vi "Shooter logic.vi"(0 "Low Pressure?":bool, 1 "Fire Main":bool, 2 "Fire 3":bool, 3 "Fire 2":bool, 5 "Grabber Button":bool, 6 "Time Between Open and Shoot":u32=250, 7 "Arms Up button":bool, 8 "Release to Retract":u32=750, 9 "Arms Down Button":bool, 10 "Arms up and down":dbl) -> ()   [LabVIEW 2013]
uses:
  <vilib>/Rock Robotics/WPI/Solenoid/WPI_SolenoidValue.ctl
  <vilib>/Rock Robotics/WPI/Solenoid/WPI_SolenoidSetEnum.vi
  Robot Global Data.vi
panel:
  in  "Arm State":enum16{"Close Arms", "Open Arms"}(ring)
  in  "Launcher State":T1(ring)
  out "Tick":u32
  out "Retract Position":T2
  out "Shooter Position":T2
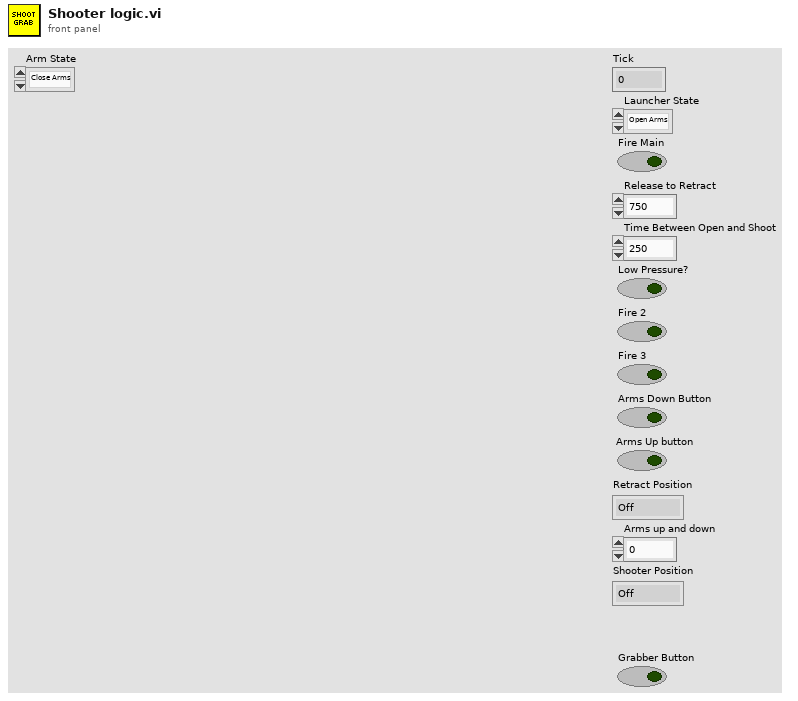
[diagram p1: front panel]
types:
  T1 = enum16{"Open Arms", "Arms Open", "Shoot", "Out", "Retract"}
  T2 = typedef "WPI_SolenoidValue.ctl" = enum16{"Off", "On", "Forward", "Reverse"}
  T3 = typedef "WPI_SolenoidDevRef.ctl" = cluster{"DevStatus":errorcluster, "Solenoid Module":T4, "Forward Solenoid Channel":T5, "Reverse Solenoid Channel":T5}
  T4 = typedef "FPGA_TypedefSolenoidModule.ctl" = enum16{"Solenoid Module 1", "Solenoid Module 2"}
  T5 = typedef "WPI_SolenoidChannel.ctl" = enum8{"Solenoid 1", "Solenoid 2", "Solenoid 3", "Solenoid 4", "Solenoid 5", "Solenoid 6", "Solenoid 7", "Solenoid 8", "Invalid"}
  T6 = typedef "WPI_DigitalInputDevRef.ctl" = cluster{"DevStatus":errorcluster, "DIO Channel":T7, "Digital Module":T8}
  T7 = typedef "FPGA_DIOChannel.ctl" = enum8{"DIO 1", "DIO 2", "DIO 3", "DIO 4", "DIO 5", "DIO 6", "DIO 7", "DIO 8", "DIO 9", "DIO 10", "DIO 11", "DIO 12", "DIO 13", "DIO 14", "Invalid"}
  T8 = typedef "FPGA_TypedefDigitalModule.ctl" = enum16{"Digital Module 1", "Digital Module 2"}
  T9 = typedef "WPI_MotorControlDeviceRef.ctl" = cluster{"DeviceStatus":errorcluster, "Type":enum16{"PWM", "CAN"}, "PWM":cluster{"Digital Module":T8, "PWM Channel":T10, "DeadBand":T11}, "CAN":cluster{"Device Number":u8, "Control Mode":T12, "Semaphore":T13, "Max Vout":dbl}, "Invert":bool, "TransformRef":T14, "InvTransformRef":T14}
  T10 = typedef "FPGA_DIOPWMChannel.ctl" = enum8{"PWM 1", "PWM 2", "PWM 3", "PWM 4", "PWM 5", "PWM 6", "PWM 7", "PWM 8", "PWM 9", "PWM 10", "Invalid"}
  T11 = typedef "WPI_PWMDeadband.ctl" = cluster{"Name":string, "maxPositivePwm":i32, "minPositivePwm":i32, "centerPwm":i32, "maxNegativePwm":i32, "minNegativePwm":i32, "angularRange":u16}
  T12 = typedef "WPI_CANJaguar_ControlMode.ctl" = enum8{"Percent VBus", "Current", "Speed", "Position", "Voltage"}
  T13 = typedef "Semaphore RefNum" = refnum<k1>
  T14 = typedef "WPI_PWMTransform_ConPane.ctl" = refnum<vi>
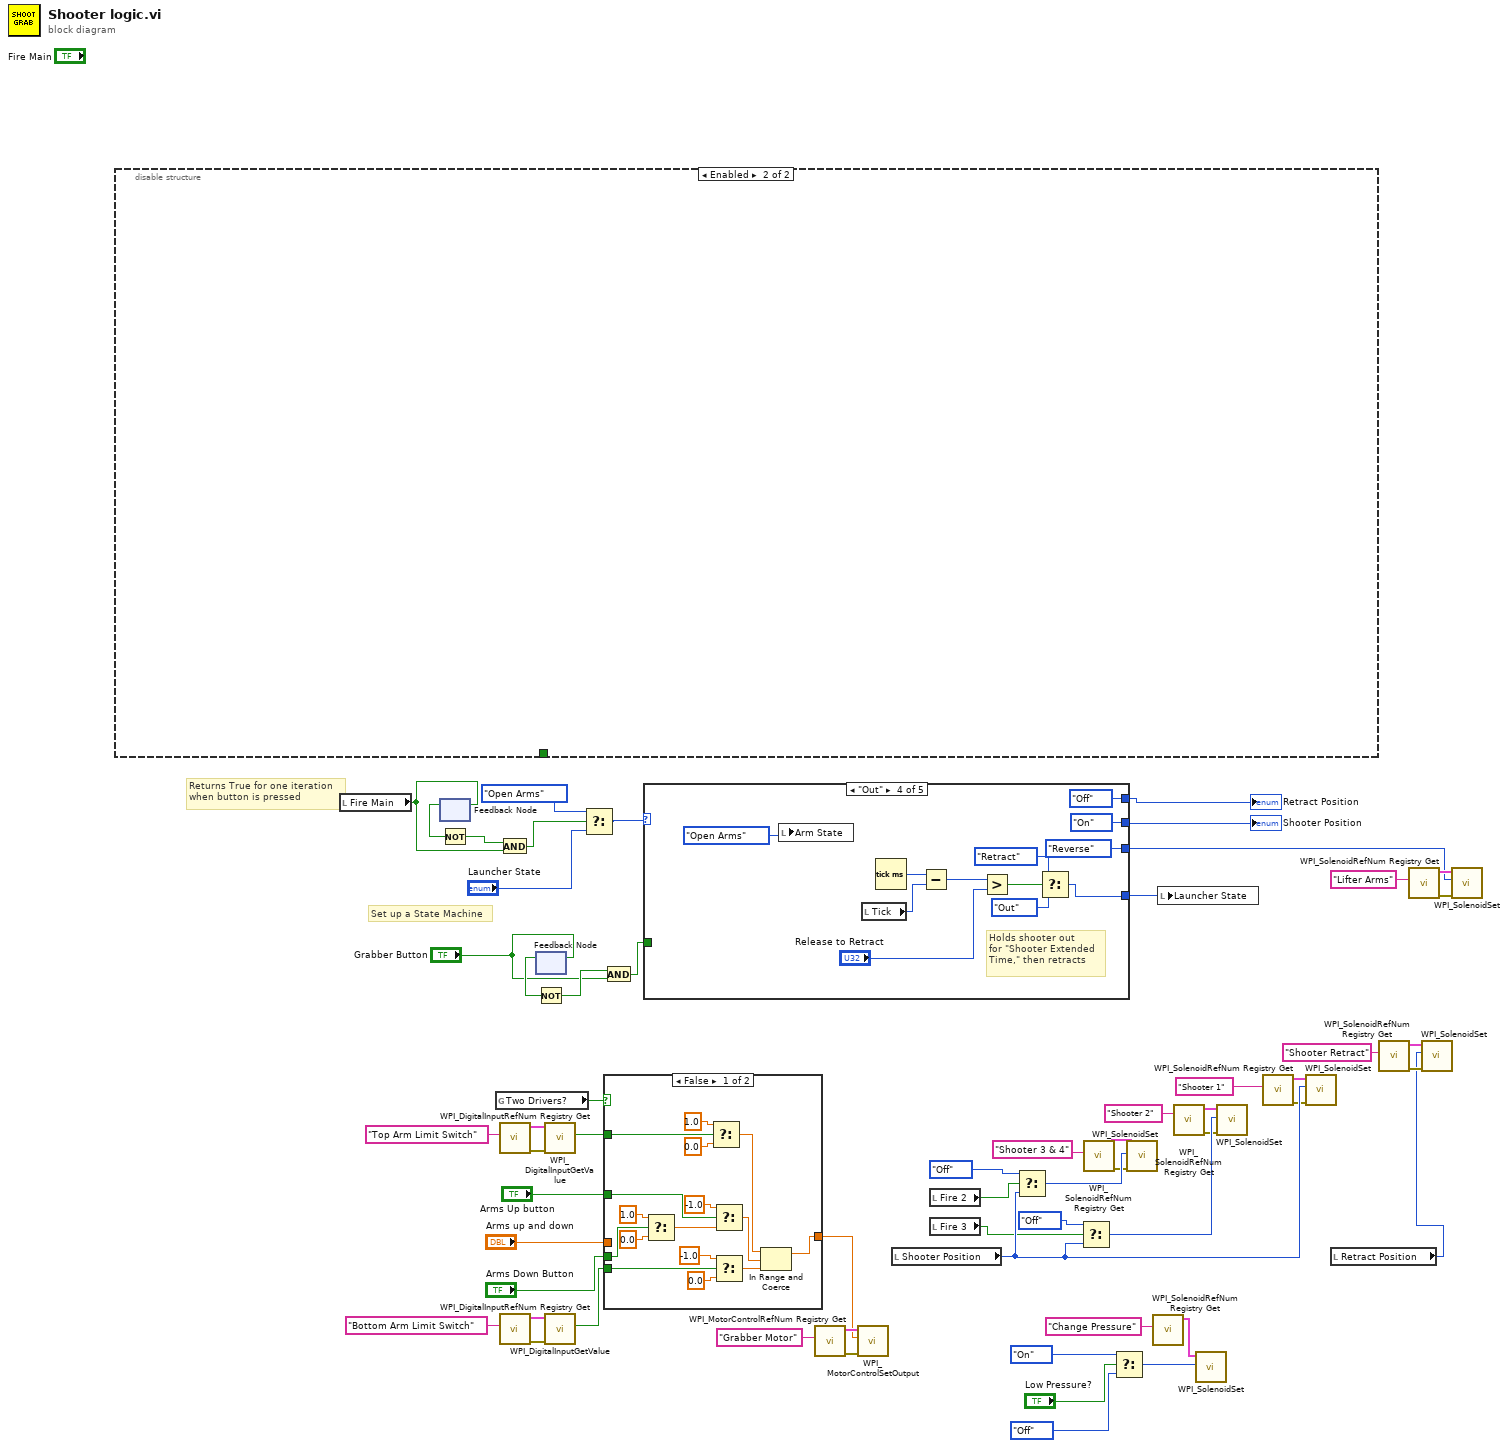
[diagram p0: block diagram]
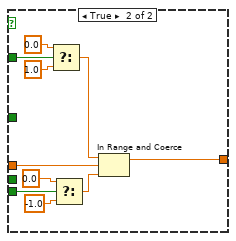
[diagram p2: hidden frame]
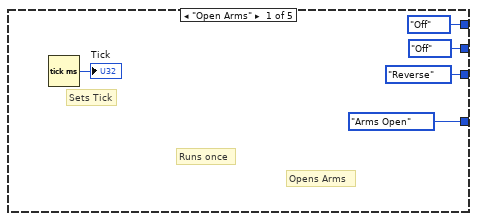
[diagram p3: hidden frame]
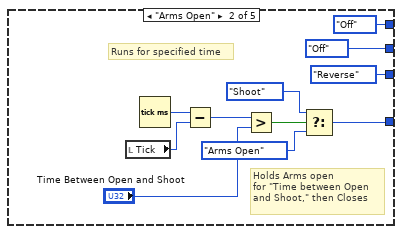
[diagram p4: hidden frame]
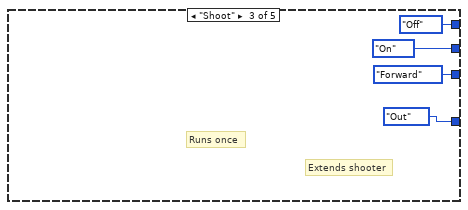
[diagram p5: hidden frame]
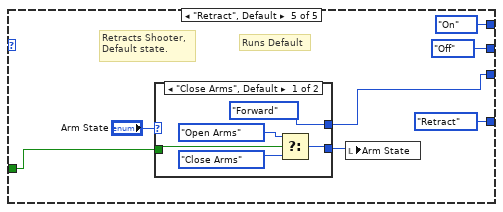
[diagram p6: hidden frame]
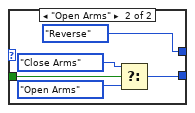
[diagram p7: hidden frame]
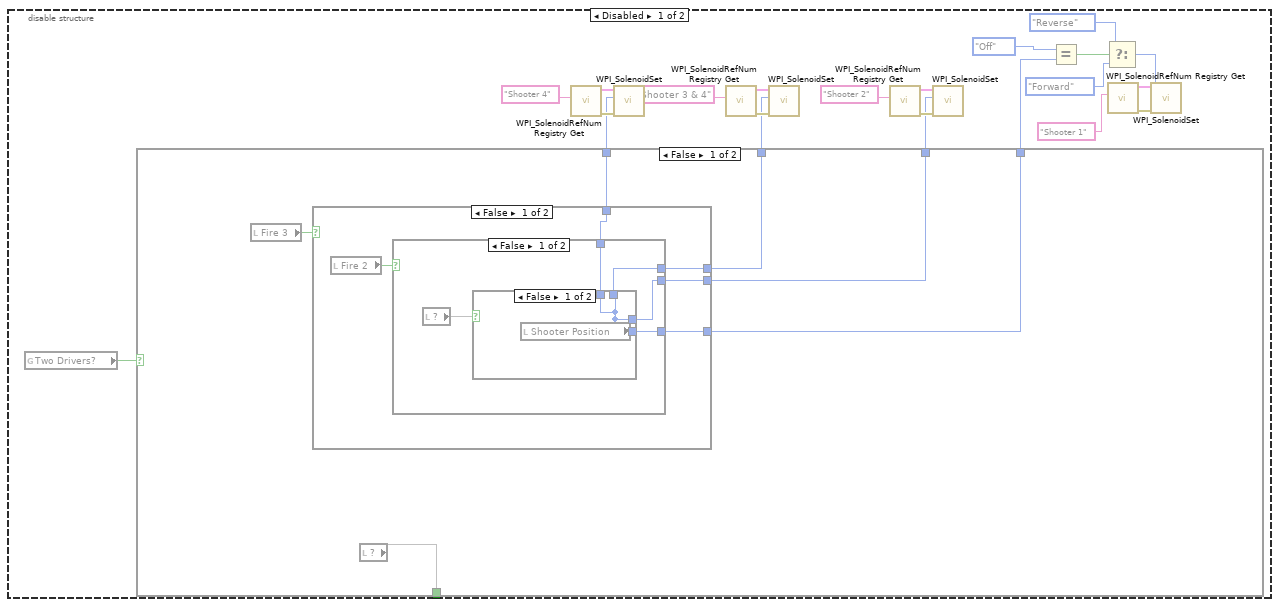
[diagram p8: hidden frame]
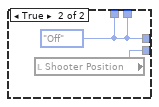
[diagram p9: hidden frame]
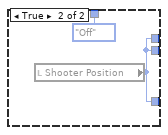
[diagram p10: hidden frame]
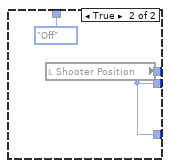
[diagram p11: hidden frame]
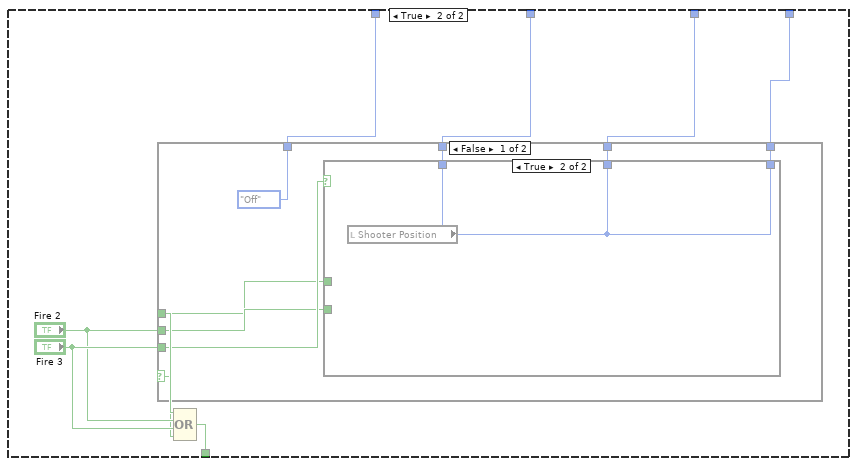
[diagram p12: hidden frame]
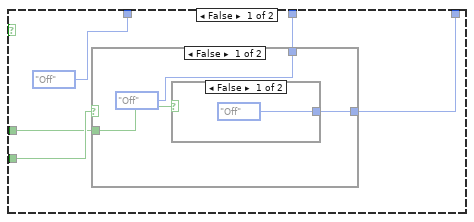
[diagram p13: hidden frame]
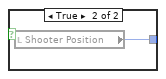
[diagram p14: hidden frame]
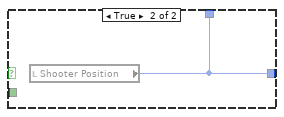
[diagram p15: hidden frame]
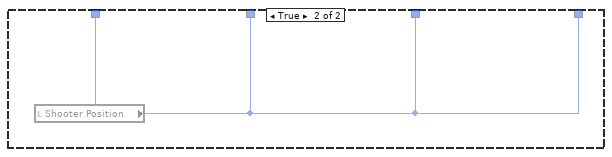
[diagram p16: hidden frame]
diagram:
  # "Set up a State Machine"
  # "Returns True for one iteration\nwhen button is pressed"
  n1 = disable-structure shown="Enabled" {
    disable-tunnel: [w83 _] -> _
    frame Disabled {
      n2 = global read "Robot Global Data.vi" "Two Drivers?"() -> (w82:bool)
      n3 = case shown="False" w82 {
        tunnel: [w89 w115] -> w83
        tunnel: [w84 w110] -> w64
        tunnel: [w87 w109] -> w63
        tunnel: [w86 w108] -> w62
        tunnel: [w85 w107] -> w61
        frame False {
          n4 = local read "Fire 3"() -> (w88:bool)
          n5 = case shown="False" w88 {
            tunnel: [w93 w106] -> w87
            tunnel: [w92 w106] -> w86
            tunnel: [w91 w106] -> w85
            tunnel: [w90 WPI_SolenoidValue."Off" ("Position")] -> w84
            frame False {
              n6 = local read "Fire 2"() -> (w94:bool)
              n7 = case shown="False" w94 {
                tunnel: [w96 w104] -> w93
                tunnel: [w97 w104] -> w92
                tunnel: [w98 w104] -> w91
                tunnel: [w95 WPI_SolenoidValue."Off" ("Position")] -> w90
                frame False {
                  n8 = local read item#-1() -> (w99)
                  n9 = case shown="False" w99 {
                    tunnel: [w100 w102] -> w98
                    tunnel: [w100 w101] -> w97
                    tunnel: [w100 w101] -> w96
                    tunnel: [w100 w101] -> w95
                    frame False {
                      n10 = local read "Shooter Position"() -> (w100:T2)
                    }
                    frame True {
                      w101 = WPI_SolenoidValue."Off" ("Position")
                      n11 = local read "Shooter Position"() -> (w102:T2)
                    }
                  }
                }
                frame True {
                  n12 = local read "Shooter Position"() -> (w104:T2)
                }
              }
            }
            frame True {
              n13 = local read "Shooter Position"() -> (w106:T2)
            }
          }
          n14 = local read item#-1() -> (w89)
        }
        frame True {
          n15 = Compound Arithmetic op=OR("Fire 2", "Fire 3") -> (w115:bool, w112:bool, w111:bool)
          n16 = case shown="False" w111 {
            tunnel: [w118 w135] -> w107
            tunnel: [w119 w135] -> w108
            tunnel: [w120 w135] -> w109
            tunnel: [WPI_SolenoidValue."Off" ("Value") w135] -> w110
            tunnel: "Fire 3" -> [w121 _]
            tunnel: "Fire 2" -> [w117 _]
            tunnel: w112 -> [w116 _]
            frame False {
              n17 = case shown="True" w121 {
                tunnel: [WPI_SolenoidValue."Off" ("Value") w134] -> w120
                tunnel: [w127 w134] -> w119
                tunnel: [w126 w134] -> w118
                tunnel: w117 -> [w125 _]
                tunnel: w116 -> [w124 _]
                frame False {
                  n18 = case shown="False" w125 {
                    tunnel: [WPI_SolenoidValue."Off" ("Value") w133] -> w127
                    tunnel: [w128 w133] -> w126
                    tunnel: w124 -> [w129 _]
                    frame False {
                      n19 = case shown="False" w129 {
                        tunnel: [WPI_SolenoidValue."Off" ("Value") w132] -> w128
                        frame False {
                        }
                        frame True {
                          n20 = local read "Shooter Position"() -> (w132:T2)
                        }
                      }
                    }
                    frame True {
                      n21 = local read "Shooter Position"() -> (w133:T2)
                    }
                  }
                }
                frame True {
                  n22 = local read "Shooter Position"() -> (w134:T2)
                }
              }
            }
            frame True {
              n23 = local read "Shooter Position"() -> (w135:T2)
            }
          }
        }
      }
      n24 = call <vilib>:"WPI_SolenoidRefNum Registry Get.vi"("refnum name"="Shooter 4") -> ("error out"=w74:errorcluster, "SolenoidDevRef"=w75:T3)  [unwired: 9 in]
      n25 = call-poly <vilib>:"WPI_SolenoidSet.vi"("error in (no error)"=w74, "Value"=w64, "SolenoidDevRef"=w75) -> ()  [unwired: 7 in, 2 out]
      n26 = call <vilib>:"WPI_SolenoidRefNum Registry Get.vi"("refnum name"="Shooter 3 & 4") -> ("error out"=w77:errorcluster, "SolenoidDevRef"=w76:T3)  [unwired: 9 in]
      n27 = call-poly <vilib>:"WPI_SolenoidSet.vi"("error in (no error)"=w77, "Value"=w63, "SolenoidDevRef"=w76) -> ()  [unwired: 7 in, 2 out]
      n28 = call <vilib>:"WPI_SolenoidRefNum Registry Get.vi"("refnum name"="Shooter 2") -> ("error out"=w80:errorcluster, "SolenoidDevRef"=w81:T3)  [unwired: 9 in]
      n29 = call-poly <vilib>:"WPI_SolenoidSet.vi"("error in (no error)"=w80, "Value"=w62, "SolenoidDevRef"=w81) -> ()  [unwired: 7 in, 2 out]
      n30 = Equal?(x=WPI_SolenoidValue."Off" ("y"), y=w61) -> (x = y?=w67:bool)
      n31 = Select(t=WPI_SolenoidValue."Reverse" ("y"), s=w67, f=WPI_SolenoidValue."Forward" ("y")) -> (s? t:f=w70:T2)
      n32 = call <vilib>:"WPI_SolenoidRefNum Registry Get.vi"("refnum name"="Shooter 1") -> ("error out"=w66:errorcluster, "SolenoidDevRef"=w65:T3)  [unwired: 9 in]
      n33 = call-poly <vilib>:"WPI_SolenoidSet.vi"("error in (no error)"=w66, "Value"=w70, "SolenoidDevRef"=w65) -> ()  [unwired: 7 in, 2 out]
    }
    frame Enabled {
    }
  }
  n34 = local read "Fire Main"() -> (w20:bool)
  n35 = feedback #1() -> (w21:bool)  [unwired: 1 in]
  n36 = feedback-in #1(w20) -> ()
  n37 = Not(x=w21) -> (.not. x?=w22:bool)
  n38 = global read "Robot Global Data.vi" "Two Drivers?"() -> (w15:bool)
  n39 = And(x=w22, y=w20) -> (x .and. y?=w17:bool)
  n40 = call <vilib>:"WPI_DigitalInputRefNum Registry Get.vi"("refnum name"="Top Arm Limit Switch") -> ("error out"=w29:errorcluster, "DigitalInputDevRef"=w30:T6)  [unwired: 9 in]
  n41 = call <vilib>:"WPI_DigitalInputRefNum Registry Get.vi"("refnum name"="Bottom Arm Limit Switch") -> ("error out"=w26:errorcluster, "DigitalInputDevRef"=w27:T6)  [unwired: 9 in]
  n42 = feedback #2() -> (w4:bool)  [unwired: 1 in]
  n43 = feedback-in #2("Grabber Button") -> ()
  n44 = Not(x=w4) -> (.not. x?=w3:bool)
  n45 = call <vilib>:"WPI_DigitalInputGetValue.vi"("error in (no error)"=w29, "DigitalInputDevRef"=w30) -> ("Value"=w14:bool)  [unwired: 7 in, 2 out]
  n46 = call <vilib>:"WPI_DigitalInputGetValue.vi"("error in (no error)"=w26, "DigitalInputDevRef"=w27) -> ("Value"=w13:bool)  [unwired: 7 in, 2 out]
  n47 = Select(t=T1."Open Arms", s=w17, f="Launcher State") -> (s? t:f=w19:T1)
  n48 = And(x=w3, y="Grabber Button") -> (x .and. y?=w1:bool)
  n49 = case shown="False" w15 {
    tunnel: w14 -> [w143 w161]
    tunnel: w13 -> [w139 w157]
    tunnel: [w136 w153] -> w10
    tunnel: "Arms Up button" -> [w138 _]
    tunnel: "Arms Down Button" -> [w137 _]
    tunnel: "Arms up and down" -> [_ w152]
    frame False {
      n50 = Select(t=1.0, s=w137, f=0.0) -> (s? t:f=w149:dbl)
      n51 = Select(t=1.0, s=w143, f=0.0) -> (s? t:f=w144:dbl)
      n52 = Select(t=-1.0, s=w138, f=w149) -> (s? t:f=w147:dbl)
      n53 = Select(t=-1.0, s=w139, f=0.0) -> (s? t:f=w140:dbl)
      n54 = In Range and Coerce(upper limit=w144, x=w147, lower limit=w140) -> (coerced(x)=w136:dbl)  [unwired: 1 out]
    }
    frame True {
      n55 = Select(t=0.0, s=w161, f=1.0) -> (s? t:f=w160:dbl)
      n56 = Select(t=0.0, s=w157, f=-1.0) -> (s? t:f=w156:dbl)
      n57 = In Range and Coerce(upper limit=w160, x=w152, lower limit=w156) -> (coerced(x)=w153:dbl)  [unwired: 1 out]
    }
  }
  n58 = case shown="\"Out\"" w19 {
    tunnel: [WPI_SolenoidValue."Off" ("Value") WPI_SolenoidValue."Off" ("Value") WPI_SolenoidValue."On" ("Value") WPI_SolenoidValue."On" ("Value") WPI_SolenoidValue."Off" ("Value")] -> w7
    tunnel: [T1."Arms Open" ("Launcher State") w168 T1."Out" ("Launcher State") w186 T1."Retract" ("Launcher State")] -> w6
    tunnel: [WPI_SolenoidValue."Reverse" ("Arm Position") WPI_SolenoidValue."Reverse" ("Arm Position") WPI_SolenoidValue."Forward" ("Arm Position") WPI_SolenoidValue."Reverse" ("Arm Position") w196] -> w5
    tunnel: [WPI_SolenoidValue."Off" ("Value") WPI_SolenoidValue."Off" ("Value") WPI_SolenoidValue."Off" ("Value") WPI_SolenoidValue."Off" ("Value") WPI_SolenoidValue."On" ("Value")] -> w8
    tunnel: w1 -> [_ _ _ _ w197]
    frame "Open Arms" {
      # "Opens Arms"
      # "Runs once"
      # "Sets Tick"
      n59 = Tick Count (ms)() -> (millisecond timer value=→"Tick":u32)
    }
    frame "Arms Open" {
      # "Runs for specified time"
      # "Holds Arms open\nfor \"Time between Open\nand Shoot,\" then Closes"
      n60 = local read "Tick"() -> (w176:u32)
      n61 = Tick Count (ms)() -> (millisecond timer value=w177:u32)
      n62 = Subtract(x=w177, y=w176) -> (x-y=w175:u32)
      n63 = Greater?(x=w175, y="Time Between Open and Shoot") -> (0:w174:bool)
      n64 = Select(t=T1."Shoot" ("Launcher State"), s=w174, f=T1."Arms Open" ("Launcher State")) -> (s? t:f=w168:T1)
    }
    frame "Shoot" {
      # "Runs once"
      # "Extends shooter"
    }
    frame "Out" {
      # "Holds shooter out\nfor \"Shooter Extended\nTime,\" then retracts"
      n65 = local write "Arm State"(enum16{"Close Arms", "Open Arms"}."Open Arms" ("Arm State")) -> ()
      n66 = local read "Tick"() -> (w192:u32)
      n67 = Tick Count (ms)() -> (millisecond timer value=w193:u32)
      n68 = Subtract(x=w193, y=w192) -> (x-y=w191:u32)
      n69 = Greater?(x=w191, y="Release to Retract") -> (0:w190:bool)
      n70 = Select(t=T1."Retract" ("Launcher State"), s=w190, f=T1."Out" ("Launcher State")) -> (s? t:f=w186:T1)
    }
    frame "Retract", Default {
      # "Runs Default"
      # "Retracts Shooter, \nDefault state."
      n71 = case shown="\"Close Arms\", Default" "Arm State" {
        tunnel: w197 -> [w201 w206]
        tunnel: [WPI_SolenoidValue."Forward" ("Value") WPI_SolenoidValue."Reverse" ("Value")] -> w196
        tunnel: [w202 w207] -> w194
        frame "Close Arms", Default {
          n72 = Select(t=enum16{"Close Arms", "Open Arms"}."Open Arms", s=w201, f=enum16{"Close Arms", "Open Arms"}."Close Arms") -> (s? t:f=w202:enum16{"Close Arms", "Open Arms"})
        }
        frame "Open Arms" {
          n73 = Select(t=enum16{"Close Arms", "Open Arms"}."Close Arms", s=w206, f=enum16{"Close Arms", "Open Arms"}."Open Arms") -> (s? t:f=w207:enum16{"Close Arms", "Open Arms"})
        }
      }
      n74 = local write "Arm State"(w194) -> ()
    }
  }
  "Shooter Position" <- w7
  "Retract Position" <- w8
  n75 = call <vilib>:"WPI_MotorControlRefNum Registry Get.vi"("refnum name"="Grabber Motor") -> ("error out"=w25:errorcluster, "MotorControlDevRef"=w24:T9)  [unwired: 9 in]
  n76 = call <vilib>:"WPI_MotorControlSetOutput.vi"("error in (no error)"=w25, "Output"=w10, "MotorControlDevRef"=w24) -> ()  [unwired: 6 in, 3 out]
  n77 = local read "Shooter Position"() -> (w57:T2)
  n78 = local read "Fire 2"() -> (w52:bool)
  n79 = local read "Fire 3"() -> (w48:bool)
  n80 = Select(t=WPI_SolenoidValue."Off", s=w52, f=w57) -> (s? t:f=w53:T2)
  n81 = Select(t=WPI_SolenoidValue."Off", s=w48, f=w57) -> (s? t:f=w49:T2)
  n82 = call <vilib>:"WPI_SolenoidRefNum Registry Get.vi"("refnum name"="Shooter 3 & 4") -> ("error out"=w43:errorcluster, "SolenoidDevRef"=w44:T3)  [unwired: 9 in]
  n83 = Select(t=WPI_SolenoidValue."On", s="Low Pressure?", f=WPI_SolenoidValue."Off" ("t")) -> (s? t:f=w34:T2)
  n84 = call-poly <vilib>:"WPI_SolenoidSet.vi"("error in (no error)"=w43, "Value"=w53, "SolenoidDevRef"=w44) -> ()  [unwired: 7 in, 2 out]
  n85 = call <vilib>:"WPI_SolenoidRefNum Registry Get.vi"("refnum name"="Change Pressure") -> ("SolenoidDevRef"=w38:T3)  [unwired: 9 in, 1 out]
  n86 = local write "Launcher State"(w6) -> ()
  n87 = call <vilib>:"WPI_SolenoidRefNum Registry Get.vi"("refnum name"="Shooter 2") -> ("error out"=w40:errorcluster, "SolenoidDevRef"=w39:T3)  [unwired: 9 in]
  n88 = call-poly <vilib>:"WPI_SolenoidSet.vi"("Value"=w34, "SolenoidDevRef"=w38) -> ()  [unwired: 8 in, 2 out]
  n89 = call-poly <vilib>:"WPI_SolenoidSet.vi"("error in (no error)"=w40, "Value"=w49, "SolenoidDevRef"=w39) -> ()  [unwired: 7 in, 2 out]
  n90 = call <vilib>:"WPI_SolenoidRefNum Registry Get.vi"("refnum name"="Shooter 1") -> ("error out"=w46:errorcluster, "SolenoidDevRef"=w47:T3)  [unwired: 9 in]
  n91 = call-poly <vilib>:"WPI_SolenoidSet.vi"("error in (no error)"=w46, "Value"=w57, "SolenoidDevRef"=w47) -> ()  [unwired: 7 in, 2 out]
  n92 = local read "Retract Position"() -> (w32:T2)
  n93 = call <vilib>:"WPI_SolenoidRefNum Registry Get.vi"("refnum name"="Shooter Retract") -> ("error out"=w55:errorcluster, "SolenoidDevRef"=w54:T3)  [unwired: 9 in]
  n94 = call <vilib>:"WPI_SolenoidRefNum Registry Get.vi"("refnum name"="Lifter Arms") -> ("error out"=w59:errorcluster, "SolenoidDevRef"=w58:T3)  [unwired: 9 in]
  n95 = call-poly <vilib>:"WPI_SolenoidSet.vi"("error in (no error)"=w55, "Value"=w32, "SolenoidDevRef"=w54) -> ()  [unwired: 7 in, 2 out]
  n96 = call-poly <vilib>:"WPI_SolenoidSet.vi"("error in (no error)"=w59, "Value"=w5, "SolenoidDevRef"=w58) -> ()  [unwired: 7 in, 2 out]
